vi "UDT_loggingModule_sendOpenLog.vi"() -> (3 "Unit Test Framework Results":T1)   [LabVIEW 2017]
doc: "Use this template to create a user-defined test VI. Define your test requirements and wire the results to the <b>Result (Test)</b> control. Do not modify the <b>Unit Test Framework Results</b> indicator."
uses:
  <vilib>/utf/common/utf_test_result_troll.ctl
  <vilib>/utf/common/utf_test_result.ctl
  <vilib>/utf/common/utf_test_result_failure.ctl
  <vilib>/utf/common/utf_test_comparison_operators.ctl
  <vilib>/utf/common/utf_vi_tag.ctl
  RT/loggingModule/Queue/TypeDefs/queueFGVState.ctl
  RT/loggingModule/loggingModule.lvlib
  <vilib>/Control Software Solutions Ltd/UTF Helper/Unit Test Helper.lvlib
  <vilib>/utf/NI_UnitTestFramework.lvlib
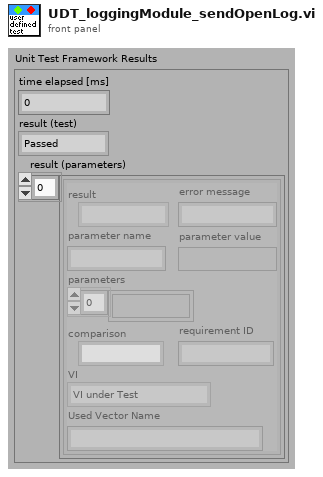
[diagram p1: front panel]
types:
  T1 = typedef "NI_UnitTestFramework.lvlib/utf_test_result_troll.ctl" = cluster{"time elapsed [ms]":u32, "result (test)":T2, "result (parameters)":T3[]}
  T2 = typedef "NI_UnitTestFramework.lvlib/utf_test_result.ctl" = enum16{"Passed", "Failed", "Error", "Skipped", "Not Processed"}
  T3 = typedef "NI_UnitTestFramework.lvlib/utf_test_result_failure.ctl" = cluster{"result":T2, "error message":string, "parameter name":string, "parameter value":variant, "parameters":variant[], "comparison":T4, "requirement ID":string, "VI":T5, "Used Vector Name":string}
  T4 = typedef "NI_UnitTestFramework.lvlib/utf_test_comparison_operators.ctl" = enum16{"=", "!=", ">", ">=", "<", "<=", "range", "symmetric tolerance", "asymmetric tolerance", "string contains", "string not contain", "array size", "string length", "array range", "by element", "array range (limit array)", "user-defined", "array contains", "array not contain", "vector length", "= (elm)", "!= (elm)", "= (case insensitive)", "!= (case insensitive)"}
  T5 = typedef "NI_UnitTestFramework.lvlib/utf_vi_tag.ctl" = enum16{"Setup VI", "VI under Test", "Teardown VI"}
  T6 = typedef "loggingModule.lvlib/queueFGVState.ctl" = enum16{"obtain", "enqueue low priority", "enqueue high priority", "dequeue", "release"}
  T7 = typedef "loggingModule.lvlib/message.ctl" = cluster{"calling module":string, "message":string, "data":variant}
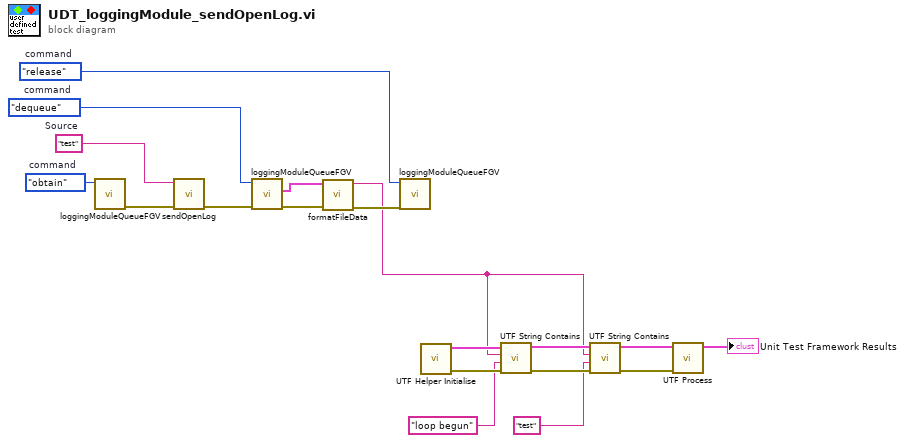
[diagram p0: block diagram]
diagram:
  w17 = queueFGVState."release"  # command
  w18 = queueFGVState."dequeue"  # command
  w4 = "test"  # Source
  w19 = queueFGVState."obtain"  # command
  n1 = call "loggingModuleQueueFGV.vi"("command"=w19) -> ("error out"=w3:errorcluster)  [unwired: 9 in, 1 out]
  n2 = call "sendOpenLog.vi"("error in (no error)"=w3, "source"=w4) -> ("error out"=w2:errorcluster)  [unwired: 9 in]
  n3 = call "loggingModuleQueueFGV.vi"("error in (no error)"=w2, "command"=w18) -> ("error out"=w10:errorcluster, "message out"=w8:T7)  [unwired: 8 in]
  n4 = call "formatFileData.vi"("error in (no error)"=w10, "message out"=w8) -> ("error out"=w9:errorcluster, "LogData"=w7:string)  [unwired: 8 in]
  n5 = call "loggingModuleQueueFGV.vi"("error in (no error)"=w9, "command"=w17) -> ()  [unwired: 8 in, 2 out]
  n6 = call <vilib>:"UTF Helper Initialise.vi"() -> ("error out"=w11:errorcluster, "results array"=w12:T3[])  [unwired: 10 in]
  n7 = call <vilib>:"UTF String Contains.vi"("error in (no error)"=w11, "Test Value"="loop begun", "Input"=w7, "Input Results"=w12) -> ("error out"=w13:errorcluster, "Output Results"=w14:T3[])  [unwired: 6 in]
  n8 = call <vilib>:"UTF String Contains.vi"("error in (no error)"=w13, "Test Value"="test", "Input"=w7, "Input Results"=w14) -> ("error out"=w16:errorcluster, "Output Results"=w15:T3[])  [unwired: 6 in]
  n9 = call <vilib>:"UTF Process.vi"("error in (no error)"=w16, "results array"=w15) -> ("Unit Test Framework Results"=→"Unit Test Framework Results":T1)  [unwired: 9 in]
